vi "dpu_read_mstr_reg.vi"(4 "str non-consec regs":u16[](array[numeric]), 5 "raw string? (n)":bool, 6 "num of str":u16=1, 7 "byte order (0:big-endian, network order)":T1(ring), 8 "error in":errorcluster, 9 "str len regs (8)":u16=8, 10 "first str reg":u16, 11 "master":refnum<class "Modbus Master.lvclass">) -> (0 "error out":errorcluster, 1 "read regs":u16[](array[numeric]), 2 "strings":string[](array[string]), 3 "master out":refnum<class "Modbus Master.lvclass">)   [LabVIEW 2014]
uses:
  protocol/modbus/ni_modbus_api/API/Master/Modbus Master.lvclass
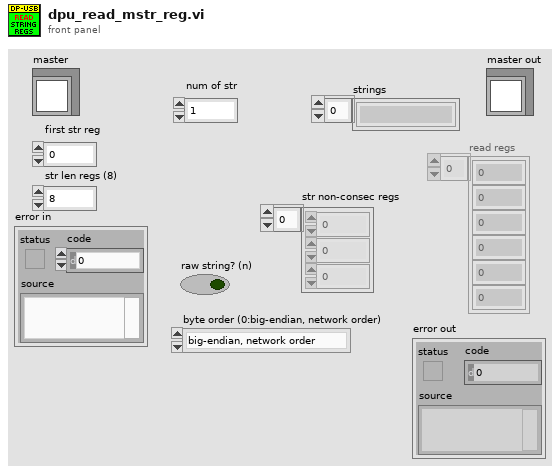
[diagram p1: front panel]
types:
  T1 = enum16{"big-endian, network order", "native, host order", "little-endian"}
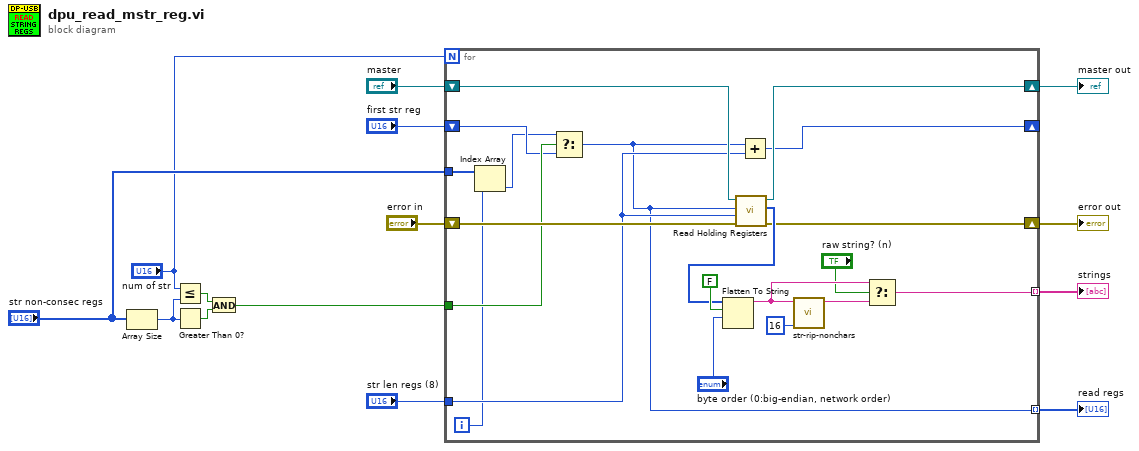
[diagram p0: block diagram]
diagram:
  n1 = Array Size(array="str non-consec regs") -> (size(s)=w9:i32)
  n2 = Less Or Equal?(x="num of str", y=w9) -> (x <= y?=w8:bool)
  n3 = Greater Than 0?(x=w9) -> (x > 0?=w7:bool)
  n4 = And(x=w8, y=w7) -> (x .and. y?=w5:bool)
  n5 = for {
    N: "num of str" -> [_]
    tunnel: "str len regs (8)" -> [w22]
    tunnel: [w25] -> w6 mode=indexing
    shift-right: [w30] -> w13
    shift-left: "master" -> [w31]
    shift-right: [w23] -> w10
    shift-left: "error in" -> [w24]
    shift-right: [w16] -> _
    shift-left: "first str reg" -> [w20]
    tunnel: w5 -> [w21]
    tunnel: "str non-consec regs" -> [w19]
    tunnel: [w15] -> w3 mode=indexing
    i -> [w18]
    n6 = Index Array(array=w19, index=w18) -> (element=w17:u16)
    n7 = Select(t=w17, s=w21, f=w20) -> (s? t:f=w15:u16)
    n8 = call-dynamic "Read Holding Registers.vi"("error in"=w24, "number of inputs"=w22, "starting address"=w15, "Modbus master in"=w31) -> ("error out"=w23:errorcluster, "register values"=w29:u16[], "Modbus master out"=w30:refnum<class "Modbus Master.lvclass">)  [unwired: 5 in]
    n9 = Flatten To String(anything=w29, prepend array or string size? (T)=FALSE, byte order (0:big-endian, network order)="byte order (0:big-endian, network order)") -> (data string=w28:string)  [unwired: 1 in, 2 out]
    n10 = Add(x=w15, y=w22) -> (x+y=w16:u16)
    n11 = call "str-rip-nonchars.vi"("clip string (0=no clipping, pos: clip, neg: clip and stop at first non printable"=16, "String_in"=w28) -> ("String_Out"=w27:string)  [unwired: 9 in]
    n12 = Select(t=w28, s="raw string? (n)", f=w27) -> (s? t:f=w25:string)
  }
  "master out" <- w13
  "error out" <- w10
  "strings" <- w6
  "read regs" <- w3
